vi "Add EngineLibs to Targets.vi"(8 "error in (no error)":errorcluster, 10 "New Library Paths":path[](array[path]), 11 "Project Sync Tools in":refnum<class "Project Sync Tools.lvclass">) -> (0 "error out":errorcluster, 3 "Project Sync Tools out":refnum<class "Project Sync Tools.lvclass">)   [LabVIEW 2019, in "Project Sync Tools.lvclass"]
uses:
  Project Sync Tools.lvclass
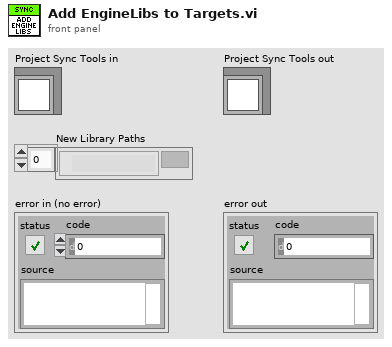
[diagram p1: front panel]
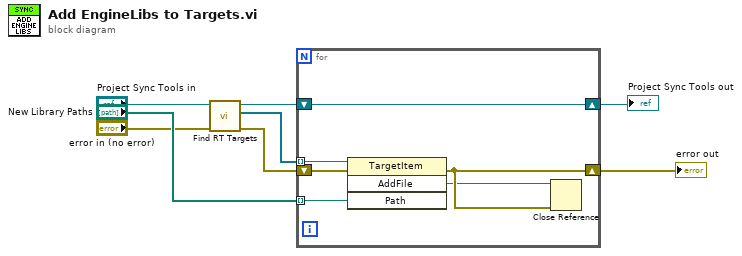
[diagram p0: block diagram]
diagram:
  n1 = call "Find RT Targets.vi"("error in (no error)"="error in (no error)", "Project Sync Tools in"="Project Sync Tools in") -> ("error out"=w5:errorcluster, "RT Targets refs"=w4:refnum<vi>[], "Project Sync Tools out"=w3:refnum<class "Project Sync Tools.lvclass">)  [unwired: 6 in, 1 out]
  n2 = for {
    tunnel: w4 -> [w14] mode=indexing
    shift-right: [w12] -> w6
    shift-left: w3 -> [w12]
    shift-right: [w11] -> w7
    shift-left: w5 -> [w13]
    tunnel: "New Library Paths" -> [w9] mode=indexing
    n3 = invoke class="TargetItem" method="AddFile"(reference=w14, error in=w13, "Path"=w9) -> (error out=w11:errorcluster, "AddFile"=w10:refnum<vi>)  [unwired: 1 in, 2 out]
    n4 = Close Reference(reference=w10, error in (no error)=w11) -> ()  [unwired: 1 out]
  }
  "error out" <- w7
  "Project Sync Tools out" <- w6
